vi "Fetch (Single).vi"(7 "Timeout (100000ms)":u32=100000, 8 "error in (no error)":errorcluster, 9 "Buffer Name ()":string, 11 "VISA resource name":refnum<visa-resource-name>) -> (0 "error out":errorcluster, 2 "Output Value":dbl, 3 "VISA resource name out":refnum<visa-resource-name>)   [LabVIEW 2023, in "Keithley DMM6500 DAQ6500 Series.lvlib"]
doc: "Read and return a measurement from the instrument. \nUse the low-level VIs for other triggering options."
uses:
  <instrlib>/Keithley DMM6500 DAQ6500 Series/Keithley DMM6500 DAQ6500 Series.lvlib
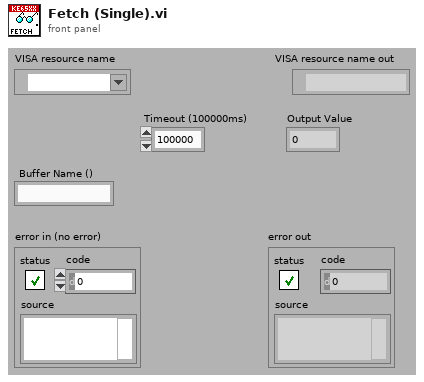
[diagram p1: front panel]
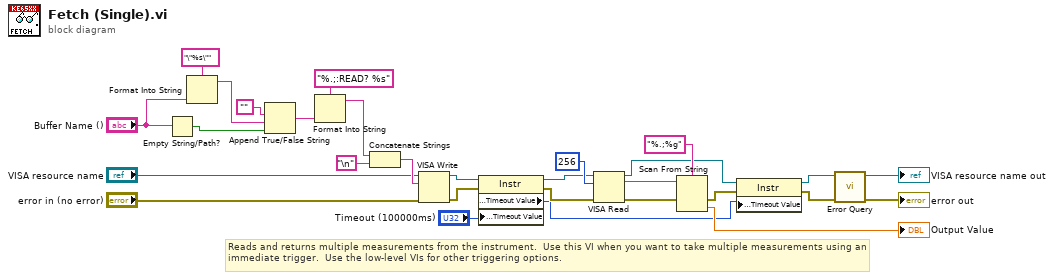
[diagram p0: block diagram]
diagram:
  # "Reads and returns multiple measurements from the instrument.  Use this VI when you want to take multiple measurements using an immediate trigger.  Use the low-level VIs for other triggering options."
  n1 = Empty String/Path?(string/path="Buffer Name ()") -> (empty?=w1:bool)
  n2 = Format Into String(format string="\"%s\"", "Buffer Name ()") -> (resulting string=w18:string)  [unwired: 2 in, 1 out]
  n3 = Append True/False String(1:w1, 2:w18, 3:"" ("Empty String Constant")) -> (0:w26:string)  [unwired: 1 in]
  n4 = Format Into String(format string="%.;:READ? %s", w26) -> (resulting string=w23:string)  [unwired: 2 in, 1 out]
  n5 = Concatenate Strings(w23, "\n" ("Line Feed Constant")) -> (w25:string)
  n6 = VISA Write(VISA resource name="VISA resource name", write buffer=w25, error in (no error)="error in (no error)") -> (VISA resource name out=w8:refnum<visa-resource-name>, error out=w6:errorcluster)  [unwired: 1 out]
  n7 = property on="Property Node" class="Instr"(reference=w8, error in=w6, "General Settings:Timeout Value"="Timeout (100000ms)") -> (reference out=w7:refnum<visa-resource-name>, error out=w5:errorcluster, "General Settings:Timeout Value"=w4:u32)
  n8 = VISA Read(VISA resource name=w7, byte count=u32 256, error in (no error)=w5) -> (VISA resource name out=w12:refnum<visa-resource-name>, read buffer=w16:string, error out=w19:errorcluster)  [unwired: 1 out]
  n9 = Scan From String(format string="%.;%g", input string=w16, error in=w19) -> (error out=w11:errorcluster, output 1=→"Output Value":dbl)  [unwired: 2 in, 2 out]
  n10 = property on="Property Node" class="Instr"(reference=w12, error in=w11, "General Settings:Timeout Value"=w4) -> (reference out=w9:refnum<visa-resource-name>, error out=w10:errorcluster)
  n11 = call <instrlib>:"Error Query.vi"("error in (no error)"=w10, "VISA resource name"=w9) -> ("error out"=→"error out":errorcluster, "VISA resource name out"=→"VISA resource name out":refnum<visa-resource-name>)  [unwired: 6 in, 2 out]
